vi "Tusk.RegisterEvent.vi"(5 "Tusk in":refnum<class "Tusk.lvclass">, 7 "error in (no error)":errorcluster, 8 "Top Level?":bool, 11 "Name (Local)":string) -> (0 "error out":errorcluster, 2 "Message Event Reg Ref":T1, 3 "Tusk out":refnum<class "Tusk.lvclass">, 4 "Tusk out (copy)":refnum<class "Tusk.lvclass">, 6 "error out (copy)":errorcluster)   [LabVIEW 2018, in "Application.lvlib" / "Tusk.lvclass"]
uses:
  Tusk.lvclass
  Message Class/Controls/Event Registration Refnum.ctl
  Message Class/Controls/User Event Reference.ctl
  Message Class/Message.lvclass
  Tusk.lvclass/Tusk.ctl
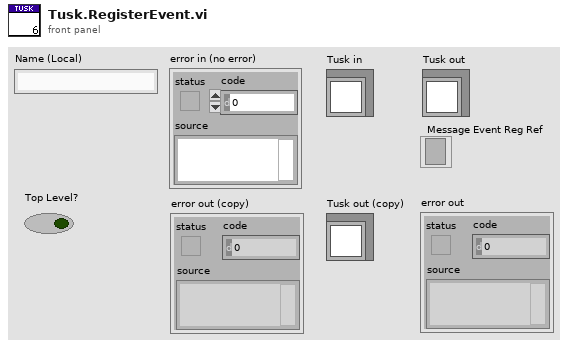
[diagram p1: front panel]
types:
  T1 = typedef "Application.lvlib/Message.lvclass/Event Registration Refnum.ctl" = refnum<event-registration>
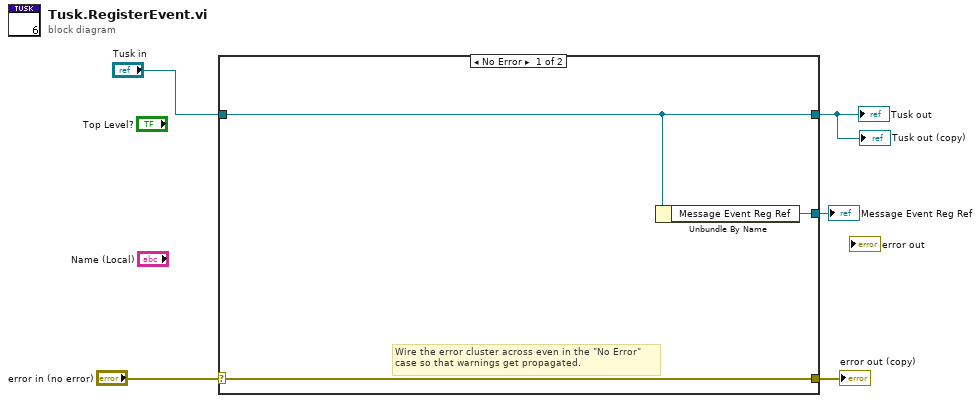
[diagram p0: block diagram]
diagram:
  n1 = case shown="No Error" "error in (no error)" {
    selector: "error in (no error)" -> [w8 w10]
    tunnel: [w8 w10] -> w4
    tunnel: [w7 w9] -> w2
    tunnel: "Tusk in" -> [w7 w9]
    tunnel: [w6 _] -> w1
    frame No Error {
      # "Wire the error cluster across even in the \"No Error\"\ncase so that warnings get propagated."
      n2 = Unbundle By Name(w7) -> ("Message Event Reg Ref"=w6:T1)
    }
    frame Error {
    }
  }
  "error out (copy)" <- w4
  "Tusk out (copy)" <- w2
  "Tusk out" <- w2
  "Message Event Reg Ref" <- w1
